vi "SizeDown.vi"() -> ()   [LabVIEW 2024, in "RefTypedCircularBuffer.Tests.Units.lvlib"]
uses:
  RefTypedCircularBuffer.Tests.Units.lvlib
  <vilib>/addons/_JKI Toolkits/Caraya/classes/Test/Test.lvclass
  <vilib>/addons/_JKI Toolkits/Caraya/classes/Assert/Assert.lvclass
  <vilib>/addons/_JKI Toolkits/Caraya/classes/Assert/Assert True.vi
  <vilib>/addons/_JKI Toolkits/Caraya/classes/Assert/Assert Equal Value_Variant.vi
  RefTypedCircularBuffer.lvclass
  TypedCircularBuffer/Type.ctl
  TypedCircularBuffer/TypedCircularBuffer.lvclass
panel:
  in  "Size down Add Expected 7":T1[](array[typedef])=[5, 6, 7, 8, 9, 10, 255]
  in  "Size down Expected 7":T1[](array[typedef])=[4, 5, 6, 7, 8, 9, 10]
  in  "Size down Add Expected 3":T1[](array[typedef])=[9, 10, 255]
  in  "Size down Expected 3":T1[](array[typedef])=[8, 9, 10]
  in  "Size down Add Expected":T1[](array[typedef])=[7, 8, 9, 10, 255]
  in  "Size down Expected":T1[](array[typedef])=[6, 7, 8, 9, 10]
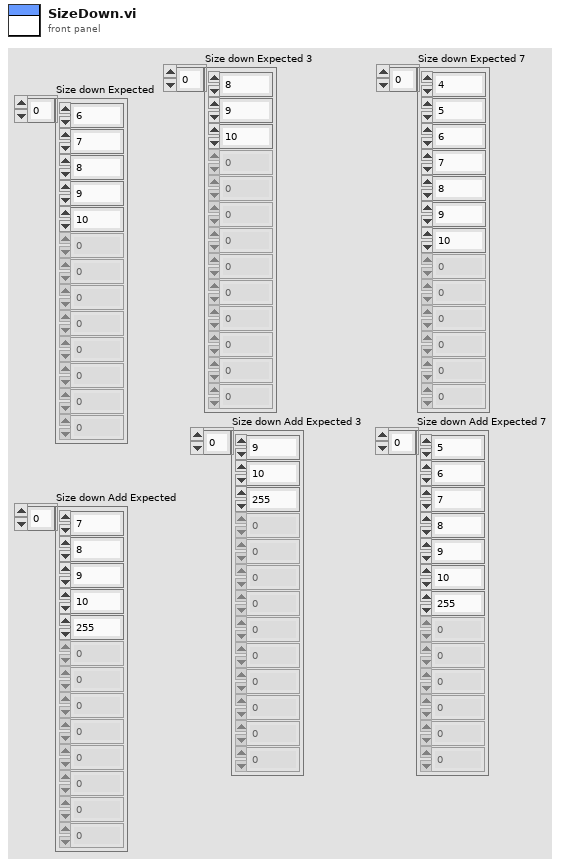
[diagram p1: front panel]
types:
  T1 = typedef "TypedCircularBuffer.lvclass/Type.ctl" = i32
  T2 = typedef "RefTypedCircularBuffer.lvclass/Type.ctl" = u8
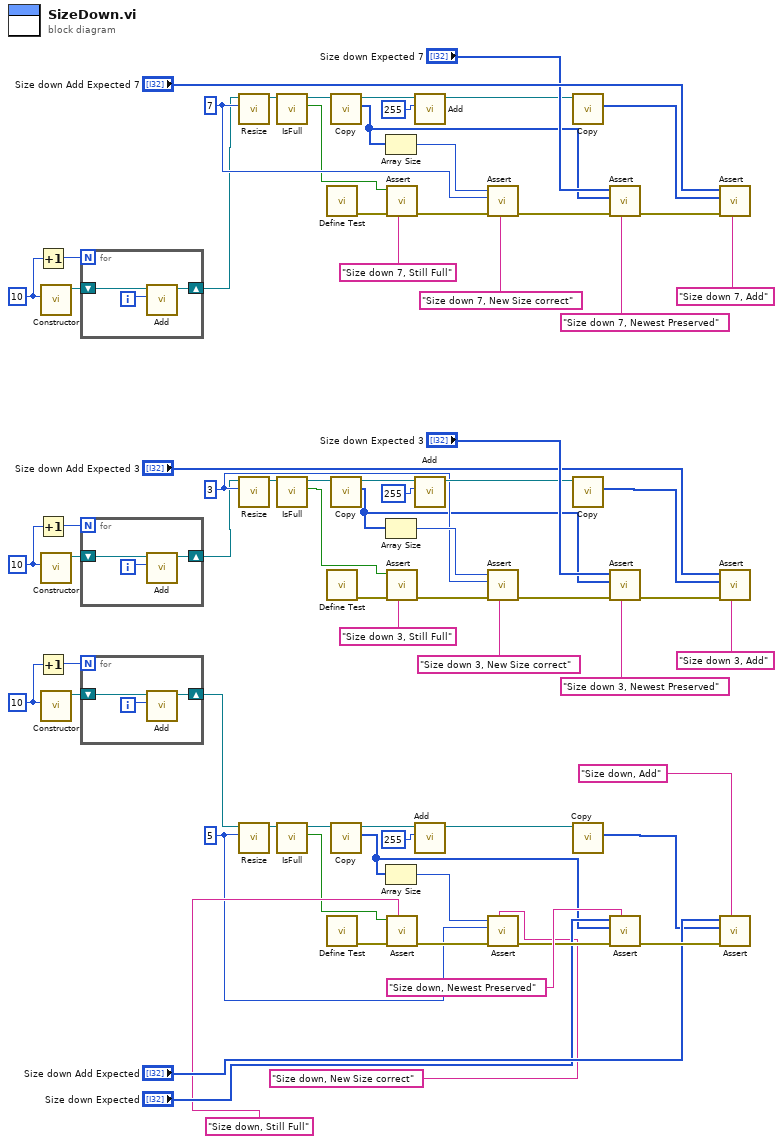
[diagram p0: block diagram]
diagram:
  w2 = u32 10 ("Capacity")
  w9 = u32 10 ("Capacity")
  w36 = u32 7 ("Capacity")
  w23 = u32 3 ("Capacity")
  w10 = u32 5 ("Capacity")
  w37 = u32 10 ("Capacity")
  n1 = Increment(x=w9) -> (x+1=w7:u32)
  n2 = Increment(x=w37) -> (x+1=w61:u32)
  n3 = Increment(x=w2) -> (x+1=w4:u32)
  n4 = call "Constructor.vi"("Capacity"=w9) -> ("TypedCircularBuffer out"=w8:refnum<class "RefTypedCircularBuffer.lvclass">)  [unwired: 10 in]
  n5 = call "Constructor.vi"("Capacity"=w37) -> ("TypedCircularBuffer out"=w38:refnum<class "RefTypedCircularBuffer.lvclass">)  [unwired: 10 in]
  n6 = call "Constructor.vi"("Capacity"=w2) -> ("TypedCircularBuffer out"=w3:refnum<class "RefTypedCircularBuffer.lvclass">)  [unwired: 10 in]
  n7 = for {
    N: w7 -> [_]
    shift-right: [w74] -> w5
    shift-left: w8 -> [w75]
    i -> [w73]
    n8 = call "Add.vi"("Element"=w73, "TypedCircularBuffer in"=w75) -> ("TypedCircularBuffer out"=w74:refnum<class "RefTypedCircularBuffer.lvclass">)  [unwired: 7 in, 2 out]
  }
  n9 = for {
    N: w61 -> [_]
    shift-right: [w77] -> w6
    shift-left: w38 -> [w78]
    i -> [w76]
    n10 = call "Add.vi"("Element"=w76, "TypedCircularBuffer in"=w78) -> ("TypedCircularBuffer out"=w77:refnum<class "RefTypedCircularBuffer.lvclass">)  [unwired: 7 in, 2 out]
  }
  n11 = for {
    N: w4 -> [_]
    shift-right: [w80] -> w1
    shift-left: w3 -> [w81]
    i -> [w79]
    n12 = call "Add.vi"("Element"=w79, "TypedCircularBuffer in"=w81) -> ("TypedCircularBuffer out"=w80:refnum<class "RefTypedCircularBuffer.lvclass">)  [unwired: 7 in, 2 out]
  }
  n13 = call "Resize.vi"("Capacity"=w36, "TypedCircularBuffer in"=w5) -> ("TypedCircularBuffer out"=w35:refnum<class "RefTypedCircularBuffer.lvclass">)  [unwired: 9 in]
  n14 = call "Resize.vi"("Capacity"=w23, "TypedCircularBuffer in"=w6) -> ("TypedCircularBuffer out"=w24:refnum<class "RefTypedCircularBuffer.lvclass">)  [unwired: 9 in]
  n15 = call "Resize.vi"("Capacity"=w10, "TypedCircularBuffer in"=w1) -> ("TypedCircularBuffer out"=w15:refnum<class "RefTypedCircularBuffer.lvclass">)  [unwired: 9 in]
  n16 = call "IsFull.vi"("TypedCircularBuffer in"=w35) -> ("Full?"=w34:bool, "TypedCircularBuffer out"=w33:refnum<class "RefTypedCircularBuffer.lvclass">)  [unwired: 9 in]
  n17 = call "IsFull.vi"("TypedCircularBuffer in"=w24) -> ("Full?"=w22:bool, "TypedCircularBuffer out"=w25:refnum<class "RefTypedCircularBuffer.lvclass">)  [unwired: 9 in]
  n18 = call "IsFull.vi"("TypedCircularBuffer in"=w15) -> ("Full?"=w11:bool, "TypedCircularBuffer out"=w16:refnum<class "RefTypedCircularBuffer.lvclass">)  [unwired: 9 in]
  n19 = call <vilib>:"Define Test.vi"() -> ("error out"=w43:errorcluster)  [unwired: 10 in, 1 out]
  n20 = call <vilib>:"Define Test.vi"() -> ("error out"=w60:errorcluster)  [unwired: 10 in, 1 out]
  n21 = call <vilib>:"Define Test.vi"() -> ("error out"=w62:errorcluster)  [unwired: 10 in, 1 out]
  n22 = call "Copy.vi"("TypedCircularBuffer in"=w33) -> ("Copied Buffer"=w28:T2[], "TypedCircularBuffer out"=w32:refnum<class "RefTypedCircularBuffer.lvclass">)  [unwired: 9 in]
  n23 = call "Copy.vi"("TypedCircularBuffer in"=w25) -> ("Copied Buffer"=w21:T2[], "TypedCircularBuffer out"=w26:refnum<class "RefTypedCircularBuffer.lvclass">)  [unwired: 9 in]
  n24 = call "Copy.vi"("TypedCircularBuffer in"=w16) -> ("Copied Buffer"=w12:T2[], "TypedCircularBuffer out"=w17:refnum<class "RefTypedCircularBuffer.lvclass">)  [unwired: 9 in]
  n25 = Array Size(array=w28) -> (size(s)=w44:i32)
  n26 = Array Size(array=w21) -> (size(s)=w58:i32)
  n27 = Array Size(array=w12) -> (size(s)=w64:i32)
  n28 = call-poly <vilib>:"Assert.vi"("Label"="Size down 7, Still Full", "error in (no error)"=w43, "True?"=w34) -> ("error out"=w45:errorcluster)  [unwired: 7 in, 1 out]
  n29 = call-poly <vilib>:"Assert.vi"("Label"="Size down 3, Still Full", "error in (no error)"=w60, "True?"=w22) -> ("error out"=w56:errorcluster)  [unwired: 7 in, 1 out]
  n30 = call-poly <vilib>:"Assert.vi"("Label"="Size down, Still Full", "error in (no error)"=w62, "True?"=w11) -> ("error out"=w66:errorcluster)  [unwired: 7 in, 1 out]
  n31 = call "Add.vi"("Element"=u8 255, "TypedCircularBuffer in"=w32) -> ("TypedCircularBuffer out"=w29:refnum<class "RefTypedCircularBuffer.lvclass">)  [unwired: 7 in, 2 out]
  n32 = call "Add.vi"("Element"=u8 255, "TypedCircularBuffer in"=w26) -> ("TypedCircularBuffer out"=w27:refnum<class "RefTypedCircularBuffer.lvclass">)  [unwired: 7 in, 2 out]
  n33 = call "Add.vi"("Element"=u8 255, "TypedCircularBuffer in"=w17) -> ("TypedCircularBuffer out"=w18:refnum<class "RefTypedCircularBuffer.lvclass">)  [unwired: 7 in, 2 out]
  n34 = call-poly <vilib>:"Assert.vi"("Label"="Size down 7, New Size correct", "error in (no error)"=w45, "Y"=w36, "X"=w44) -> ("error out"=w46:errorcluster)  [unwired: 6 in, 1 out]
  n35 = call-poly <vilib>:"Assert.vi"("Label"="Size down 3, New Size correct", "error in (no error)"=w56, "Y"=w23, "X"=w58) -> ("error out"=w55:errorcluster)  [unwired: 6 in, 1 out]
  n36 = call-poly <vilib>:"Assert.vi"("Label"="Size down, New Size correct", "error in (no error)"=w66, "Y"=w10, "X"=w64) -> ("error out"=w68:errorcluster)  [unwired: 6 in, 1 out]
  n37 = call "Copy.vi"("TypedCircularBuffer in"=w29) -> ("Copied Buffer"=w30:T2[])  [unwired: 9 in, 1 out]
  n38 = call "Copy.vi"("TypedCircularBuffer in"=w27) -> ("Copied Buffer"=w19:T2[])  [unwired: 9 in, 1 out]
  n39 = call "Copy.vi"("TypedCircularBuffer in"=w18) -> ("Copied Buffer"=w14:T2[])  [unwired: 9 in, 1 out]
  n40 = call-poly <vilib>:"Assert.vi"("Label"="Size down 7, Newest Preserved", "error in (no error)"=w46, "Y"=w28, "X"="Size down Expected 7") -> ("error out"=w47:errorcluster)  [unwired: 6 in, 1 out]
  n41 = call-poly <vilib>:"Assert.vi"("Label"="Size down 3, Newest Preserved", "error in (no error)"=w55, "Y"=w21, "X"="Size down Expected 3") -> ("error out"=w52:errorcluster)  [unwired: 6 in, 1 out]
  n42 = call-poly <vilib>:"Assert.vi"("Label"="Size down, Newest Preserved", "error in (no error)"=w68, "Y"=w12, "X"="Size down Expected") -> ("error out"=w72:errorcluster)  [unwired: 6 in, 1 out]
  n43 = call-poly <vilib>:"Assert.vi"("Label"="Size down 7, Add", "error in (no error)"=w47, "Y"=w30, "X"="Size down Add Expected 7") -> ()  [unwired: 6 in, 2 out]
  n44 = call-poly <vilib>:"Assert.vi"("Label"="Size down 3, Add", "error in (no error)"=w52, "Y"=w19, "X"="Size down Add Expected 3") -> ()  [unwired: 6 in, 2 out]
  n45 = call-poly <vilib>:"Assert.vi"("Label"="Size down, Add", "error in (no error)"=w72, "Y"=w14, "X"="Size down Add Expected") -> ()  [unwired: 6 in, 2 out]
